vi "Config to String.vi"(11 "Gas Sequence":T1[](array[typedef])) -> (3 "Gas":string[][](array[string]))   [LabVIEW 2015]
uses:
  Tests/Controls/Gas Info.ctl
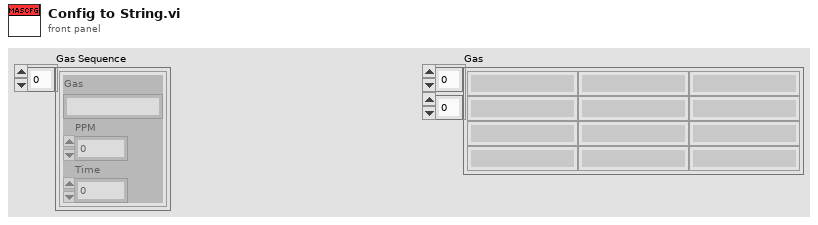
[diagram p1: front panel]
types:
  T1 = typedef "Gas Info.ctl" = cluster{"Gas":string, "PPM":dbl, "Time":u32}
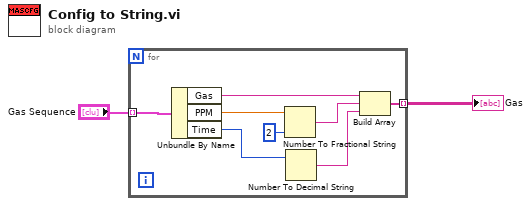
[diagram p0: block diagram]
diagram:
  n1 = for {
    tunnel: [w7] -> w2 mode=indexing
    tunnel: "Gas Sequence" -> [w6] mode=indexing
    n2 = Unbundle By Name(w6) -> ("Gas"=w10:string, "PPM"=w9:dbl, "Time"=w4:u32)
    n3 = Number To Fractional String(number=w9, precision (6)=i16 2) -> (F-format string=w8:string)  [unwired: 2 in]
    n4 = Number To Decimal String(number=w4) -> (decimal integer string=w3:string)  [unwired: 1 in]
    n5 = Build Array(w10, w8, w3) -> (w7:string[])
  }
  "Gas" <- w2
